vi "Test_Tank_Control.vi"() -> ()   [LabVIEW 2024]
doc: "This example performs writes and reads on a serial port, as directed by the user. You can press the Write and Read buttons, and change the Read Count, while the example is running.\n\nThe parameters set for the serial port must match the parameters of the connected instrument or device. In this example, the Read Count parameter specifies the number of bytes that the serial port reads. If there were more bytes at the port than the specified number, those bytes would not be read. If there were less bytes at the port than the specified number, you would receive a timeout error.\n\nThis example expands upon the flow control options for XON and XOFF, allowing the user to choose those control characters. Also, the user can enable or disable a termination character. Some devices require a termination character in order to identify the end of command strings. Some devices send a termination character to signify the end of data to be read. This example shows how you can end the Read operation once a termination character is detected in the buffer and/or append a termination character at the end of the Write data."
uses:
  LabVIEW_InstrDriver_forLK-G3000_ver1_0_1_0/32bit/Keyence LK-G3000/Public/clusters/LKIF_FLOATVALUE.ctl
  LabVIEW_InstrDriver_forLK-G3000_ver1_0_1_0/32bit/Keyence LK-G3000/Public/enums/LKIF_FLOATRESULT.ctl
  <vilib>/Instr/_visa.llb/VISA Configure Serial Port (Instr).vi
  LabVIEW_InstrDriver_forLK-G3000_ver1_0_1_0/32bit/Keyence LK-G3000/Keyence LK-G3000.lvlib
panel:
  out "Va":sgl
  out "Vb":sgl
  out "CalcData2":T1 {"LKIF_FLOATRESULT" items=["VALID", "RANGEOVER_P", "RANGEOVER_N", "WAITING"]}
  out "CalcData1":T1 {"LKIF_FLOATRESULT" items=["VALID", "RANGEOVER_P", "RANGEOVER_N", "WAITING"]}
  out "Trend Graph":cluster{"Value":sgl, "Value":sgl}(graph)
  out "Read Buffer":string[](array[string])
  in  "DRAIN":bool
  in  "FILL":bool
  in  "Stop Button":bool
  in  "State":enum16{"INIT", "IDLE", "STOP", "FILL", "DRAIN"}(ring)
  in  "2108 CDC Virtual COM":refnum<visa-resource-name>="COM3"
  # "Analog In\n\nencode 0\nslist 0 0\nslist 1 1\nsrate 6000\nps 2\ndec 1\ndeca 3\nnop"
  # "encode 0\nslist 0 0\nslist 1 1\nsrate 6000\nps 2\ndec 1\ndeca 3\nnop"
  # "encode 0 Enables the binary output mode (DEFAULT"
  # "info 0    Returns \"info 0 DATAQ\"\ninfo 1    Returns device model number (e.g.\"info 1 2008\")\ninfo 2    Returns firmware revision, 2 hex bytes (e.g. 6516 = 10110 for firmware revision 1.01)\ninfo 3    to info 4 Proprietary internal use for initial system verification\ninfo 5    <arg0>\n            Sets device description string arg0 (31 characters followed by null). Issued without <arg0> returns the \n            previously defined device description string. arg0 may be contained within quotation marks to included spaces \n            in device description. Model DI-2008 does not support info 5.\ninfo 6    Returns the instrument's serial number (left-most 8 digits only)\ninfo 7    to info 8 Proprietary internal use for initial system verification\ninfo 9    Returns the sample rate dividend value based upon current settings (see the srate command for details"
  # "0x60 = 96   FILL\n0x40 = 64  OFF\n0x20 = 32  DRAIN\n0x00 = 00  OFF"
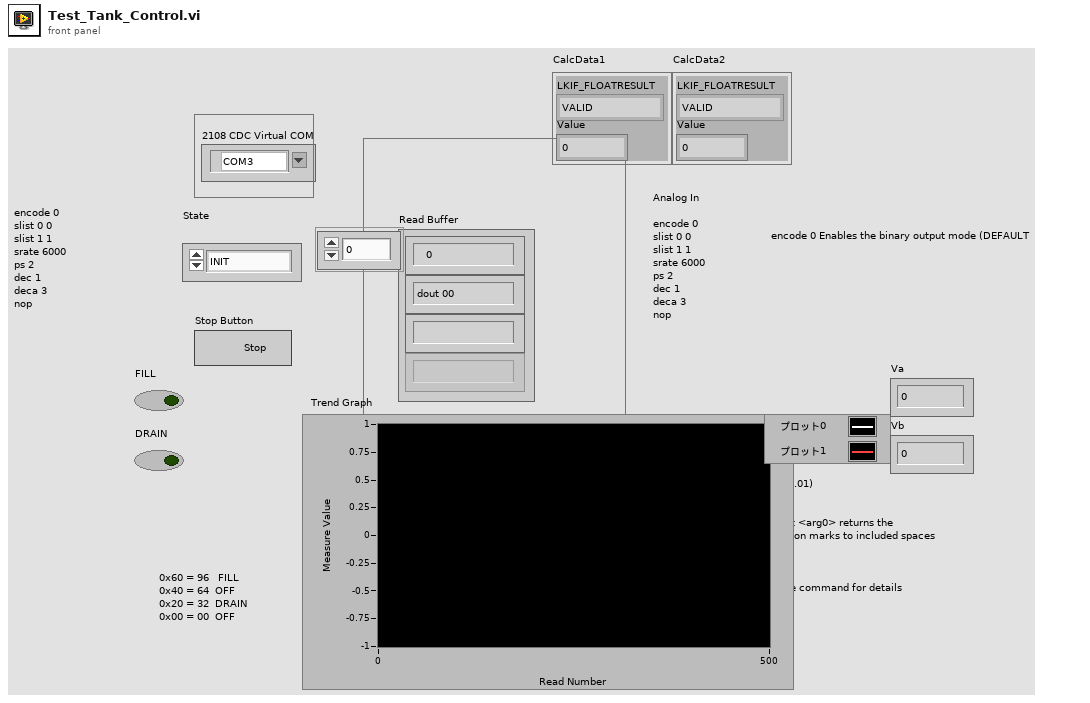
[diagram p1: front panel]
types:
  T1 = typedef "Keyence LK-G3000.lvlib/LKIF_FLOATVALUE.ctl" = cluster{"LKIF_FLOATRESULT":T2, "Value":sgl}
  T2 = typedef "Keyence LK-G3000.lvlib/LKIF_FLOATRESULT.ctl" = i32
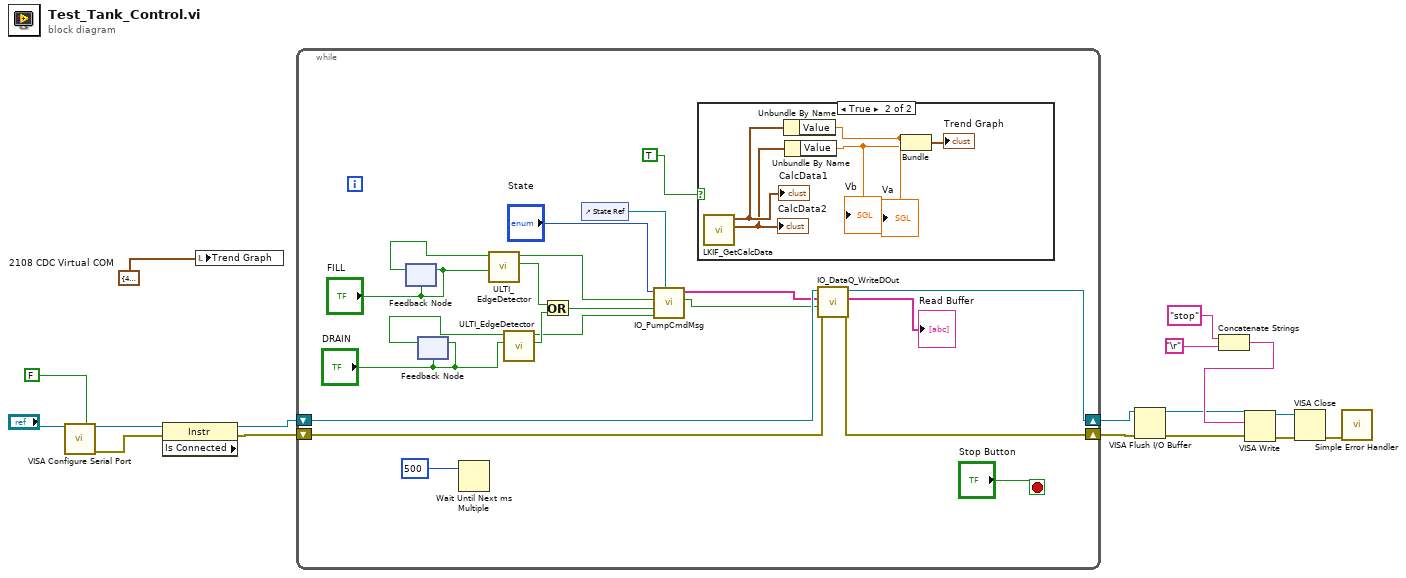
[diagram p0: block diagram]
diagram:
  n1 = call-poly "VISA Configure Serial Port"("VISA resource name"="2108 CDC Virtual COM", "Enable Termination\nChar (T)"=FALSE) -> ("VISA resource name out"=w15:refnum<visa-resource-name>, "error out"=w17:errorcluster)  [unwired: 8 in, 4 out]
  n2 = property class="Instr" props=["Is Connected"](reference=w15, error in=w17) -> (reference out=w5:refnum<visa-resource-name>, error out=w4:errorcluster)  [unwired: 1 out]
  n3 = local write "Trend Graph"(cluster{"Value":sgl, "Value":sgl} {"Value"=4.6782, "Value"=4678.4} ("Trend Graph")) -> ()
  n4 = while {
    shift-right: [w38] -> w7
    shift-left: w5 -> [w36]
    shift-right: [w37] -> w6
    shift-left: w4 -> [w35]
    stop <- "Stop Button" stop-if-true
    n5 = feedback #1("FILL") -> (w27:bool)
    n6 = feedback-in #1("FILL") -> ()
    n7 = feedback #2("DRAIN") -> (w29:bool)
    n8 = feedback-in #2("DRAIN") -> ()
    n9 = Wait Until Next ms Multiple(millisecond multiple=500) -> ()  [unwired: 1 out]
    n10 = call "ULTI_EdgeDetector.vi"("IN (N)"="FILL", "IN (N+2)"=w27) -> ("Neg Edge"=w24:bool, "Pos Edge"=w23:bool)  [unwired: 8 in]
    n11 = call "ULTI_EdgeDetector.vi"("IN (N)"="DRAIN", "IN (N+2)"=w29) -> ("Neg Edge"=w22:bool, "Pos Edge"=w21:bool)  [unwired: 8 in]
    n12 = Or(x=w24, y=w22) -> (x .or. y?=w25:bool)
    n13 = control-ref of="State Ref"() -> (w19:refnum<vi>)
    n14 = call "IO_PumpCmdMsg.vi"("State Ref"=w19, "Drain Signal"=w21, "Stop Signal"=w25, "FIll Signal"=w23, "State\n in"="State") -> ("Msg Active"=w34:bool, "Message"=w31:string[])  [unwired: 5 in]
    n15 = case shown="True" TRUE {
      frame False {
      }
      frame True {
        n16 = call "LKIF_GetCalcData.vi"() -> ("CalcData2"=w42:T1, "CalcData1"=w43:T1)  [unwired: 9 in, 1 out]
        "CalcData1" <- w43
        "CalcData2" <- w42
        n17 = Unbundle By Name(w43) -> ("Value"=w41:sgl)
        "Va" <- w41
        n18 = Unbundle By Name(w42) -> ("Value"=w40:sgl)
        "Vb" <- w40
        n19 = Bundle("Value"=w41, "Value"=w40) -> (→"Trend Graph":cluster{"Value":sgl, "Value":sgl})  [unwired: 1 in]
      }
    }
    n20 = call "IO_DataQ_WriteDOut.vi"("error in (no error)"=w35, "Msg Active"=w34, "Message"=w31, "VISA Refnum in"=w36) -> ("error out"=w37:errorcluster, "Read Buffer"=→"Read Buffer":string[], "VISA Refnum out"=w38:refnum<visa-resource-name>)  [unwired: 5 in]
  }
  n21 = VISA Flush I/O Buffer(VISA resource name=w7, error in (no error)=w6) -> (VISA resource name out=w3:refnum<visa-resource-name>, error out=w2:errorcluster)  [unwired: 1 in]
  n22 = Concatenate Strings("stop", "\r") -> (w9:string)
  n23 = VISA Write(VISA resource name=w3, write buffer=w9, error in (no error)=w2) -> (VISA resource name out=w13:refnum<visa-resource-name>, error out=w12:errorcluster)  [unwired: 1 out]
  n24 = VISA Close(VISA resource name=w13, error in (no error)=w12) -> (error out=w16:errorcluster)
  n25 = call <vilib>:"Simple Error Handler.vi"("error in (no error)"=w16) -> ()  [unwired: 1 in, 8 out]
